vi "Write Status Source.vi"(8 "error in (no error)":errorcluster, 10 "Status Source":T1, 11 "DeviceComms in":refnum<class "DeviceComms.lvclass">) -> (0 "error out":errorcluster, 3 "DeviceComms out":refnum<class "DeviceComms.lvclass">)   [LabVIEW 2024, in "CTI.lvlib" / "DeviceComms.lvclass"]
uses:
  DeviceComms.lvclass
  Status Source.ctl
  CTI.lvlib
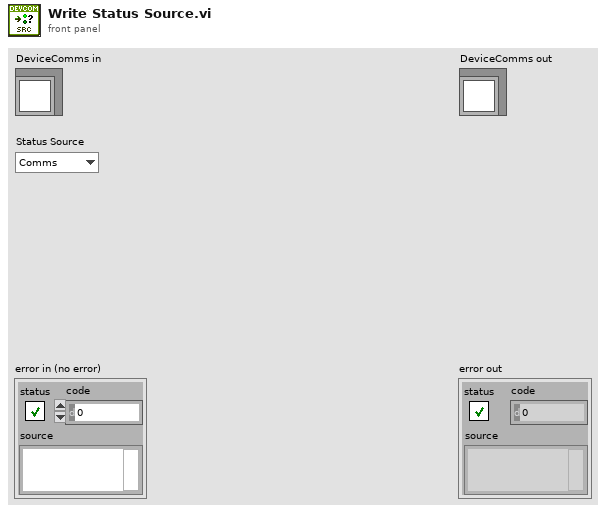
[diagram p1: front panel]
types:
  T1 = typedef "CTI.lvlib/Status Source.ctl" = enum16{"Comms", "User"}
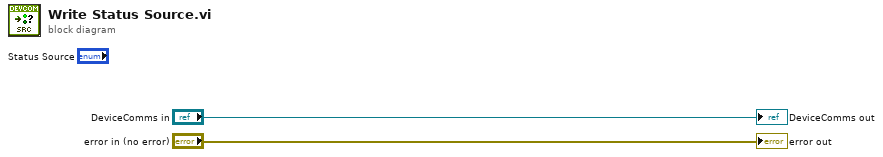
[diagram p0: block diagram]
diagram:
  "error out" <- "error in (no error)"
  "DeviceComms out" <- "DeviceComms in"
